vi "Prep Stage.vi"(8 "error in (no error)":errorcluster, 11 "Recipe Process in":refnum<class "Recipe Process.lvclass">) -> (0 "error out":errorcluster, 3 "Recipe Process out":refnum<class "Recipe Process.lvclass">)   [LabVIEW 2022 SP3, in "Recipe Process.lvlib" / "Recipe Process.lvclass"]
uses:
  Recipe Process.lvclass
  Recipe Process.lvclass/Recipe Process.ctl
  XY Stage/Interfaces/2-Axis Stage API/2-Axis Stage Async API.lvclass
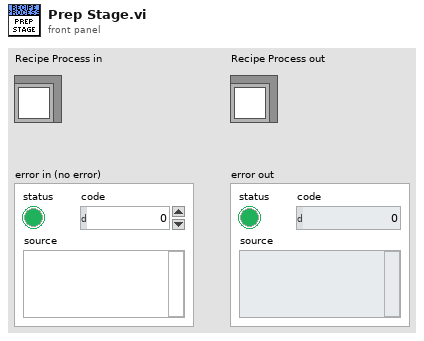
[diagram p1: front panel]
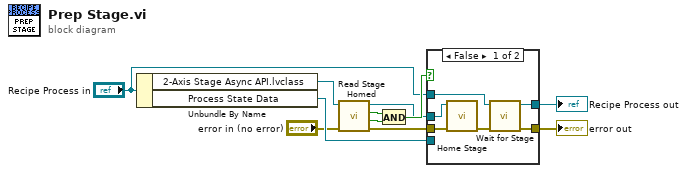
[diagram p0: block diagram]
diagram:
  n1 = Unbundle By Name("Recipe Process in") -> ("2-Axis Stage Async API.lvclass"=w11:refnum<class "2-Axis Stage Async API.lvclass">, "Process State Data"=w5:refnum<data-value>)
  n2 = call-dynamic "Read Stage Homed.vi"("error in (no error)"="error in (no error)", "2-Axis Stage Status in"=w11) -> ("error out"=w6:errorcluster, "Y-Axis Homed"=w9:bool, "X-Axis Homed"=w10:bool, "2-Axis Stage Status out"=w7:refnum<class "2-Axis Stage Async API.lvclass">)  [unwired: 6 in]
  n3 = And(x=w10, y=w9) -> (x .and. y?=w8:bool)
  n4 = case shown="False" w8 {
    tunnel: w7 -> [w17 _]
    tunnel: w6 -> [w16 w19]
    tunnel: w5 -> [_ _]
    tunnel: [w14 w19] -> w3
    tunnel: "Recipe Process in" -> [w13 w18]
    tunnel: [w12 w18] -> w1
    frame False {
      n5 = call-dynamic "Home Stage.vi"("error in (no error)"=w16, "2-Axis Async Home in"=w17) -> ("error out"=w15:errorcluster)  [unwired: 8 in, 1 out]
      n6 = call "Wait for Stage.vi"("error in (no error)"=w15, "Recipe Process in"=w13) -> ("error out"=w14:errorcluster, "Recipe Process out"=w12:refnum<class "Recipe Process.lvclass">)  [unwired: 8 in]
    }
    frame True {
    }
  }
  "Recipe Process out" <- w1
  "error out" <- w3
